vi "Get_Preset_File.vi"() -> ()   [LabVIEW 2020]
uses:
  Shared/MySQL/Preset Query Enum.ctl
panel:
  in  "Tab Control":enum32{" MAIN", "Page 2"}(tab)
  in  "Upload as Preset":bool
  in  "Preset Menu":u16(ring) items=["None", "Pulsed Alignment", "3J", "Diode", "26J", "SingleShot", "1Hz", "800 MAX ND", "Amp3-8J-CapExit", "SDI", "CapInHexPosition", "CapOutHexFiberPosition", "Full Heater, Frog Out", "Full Heater, Frog In", "MagSpecSimulateBoff", "Pulsed", "CW", "Amp2, Clunker In", "Amp3-17J", "MagSpecSimulateBon", "SMFiber-In", "SMFiber-Out", "Amp3-MegaAttenuator", "developer"]
  in  "View Preset":bool
  in  "Load ECS to Table":bool
  in  "file (use dialog)":path
  in  "Table Control":string[][](table)
  in  "Choose Values":bool
  in  "EXIT":bool
  in  "Left Join":bool
  out "PRESET FROM DB":string[][](table)
  out "ECS File":string[][](table)
  out "Coordinate Array":i32[][](array[numeric])
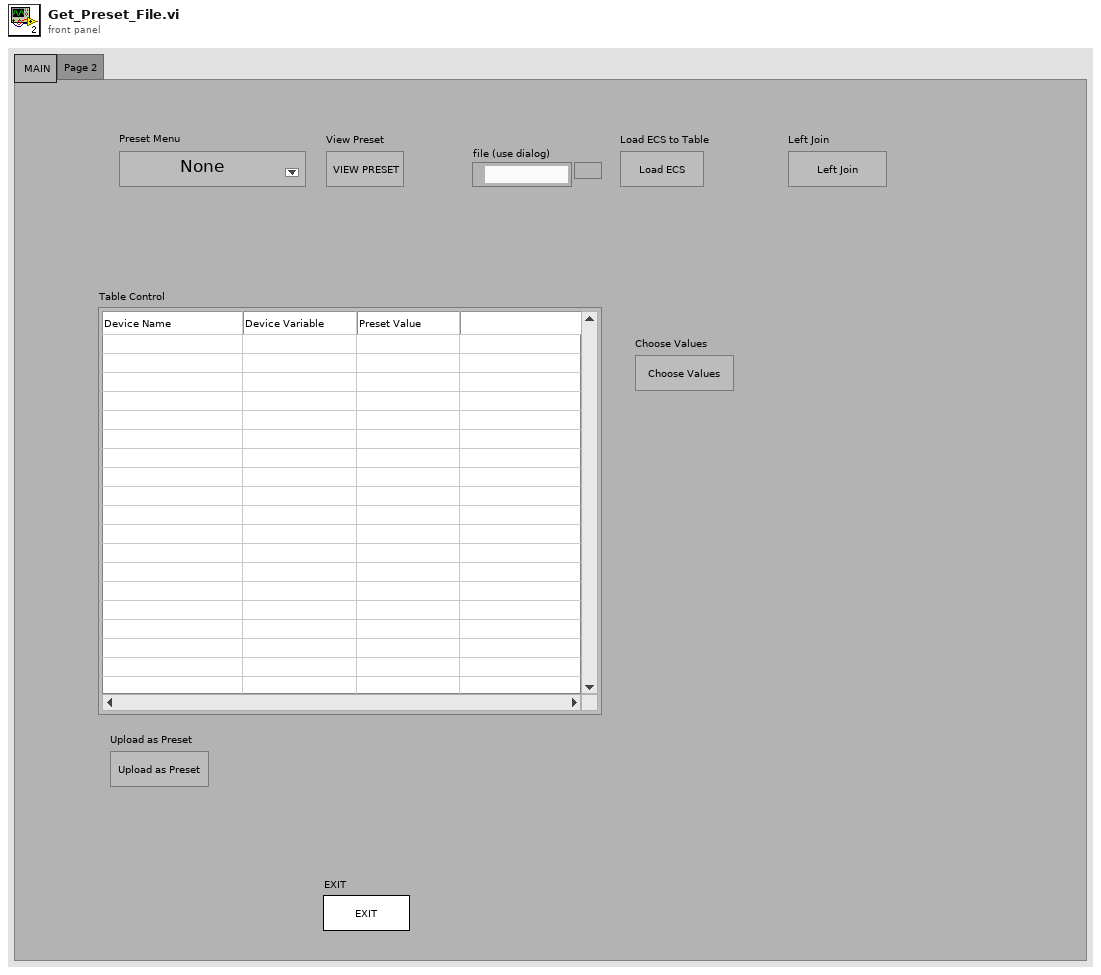
[diagram p1: front panel]
types:
  T1 = typedef "Preset Query Enum.ctl" = enum16{"Get Locations", "Get all IPs and MACs", "Get classes", "Get expt variables to set at scanstart for particular device", "Get expt devices and variables with start values", "Get expt devices and variables (with data to get)", "Get expt devices with data to get", "Get Expt devices and GUIs", "Get all devices basic properties", "Get Virtual Devices Core Info", "Get Expt names", "Get experiment basic properties", "Get experiment alarm variables", "Get MC Ports", "Get device network comm port", "Get devicetype lvclass path", "Get basic device properties", "Get Init Order", "Get all setable variables of a device", "Get device variable aliases", "Get force values of all settable variables", "Get all variables of a devicetype", "Get all variables of a device", "Get plotter details", "Get Saved Scans", "Get Scan Info", "GetGeneralGUIs", "Get expt for plotter", "Get plotter IDs from expt", "Get all devices", "Get all Virtual Devices", "Get all aliases", "Get variable and device info for Virtual Device", "GetItemLocatorIP", "Get IPs for GUIs", "Get DeviceType from Device", "GetLocalPortRange", "GetDevicePresetVariables", "Get Device Configuration", "GetAllPresetNames", "GetAllConfigurationNames", "GetPresetDeviceNames", "GetDeviceAliases", "GetDevicesOfClass"}
  T2 = enum32{"Invalid", "Standard", "Closed", "Hidden", "Minimized", "Maximized"}
  T3 = enum32{"invalid app kind", "Development System", "Run Time System", "Student Edition", "Embedded LabVIEW", "Evaluation", "Custom"}
  T4 = cluster{"Core":cluster{"Current VI Reference":refnum<vi>, "Close Panel on Exit?":bool}, "Your Boolean data":bool, "Your string data":string, "Table Control":string[][], "Column Headers[]":string[], "Temporary Preset":string[][]}
  T5 = cluster{"Current VI Reference":refnum<vi>, "Close Panel on Exit?":bool}
  T6 = enum16{"Left Button", "Center Button", "Right Button", "Window Close"}
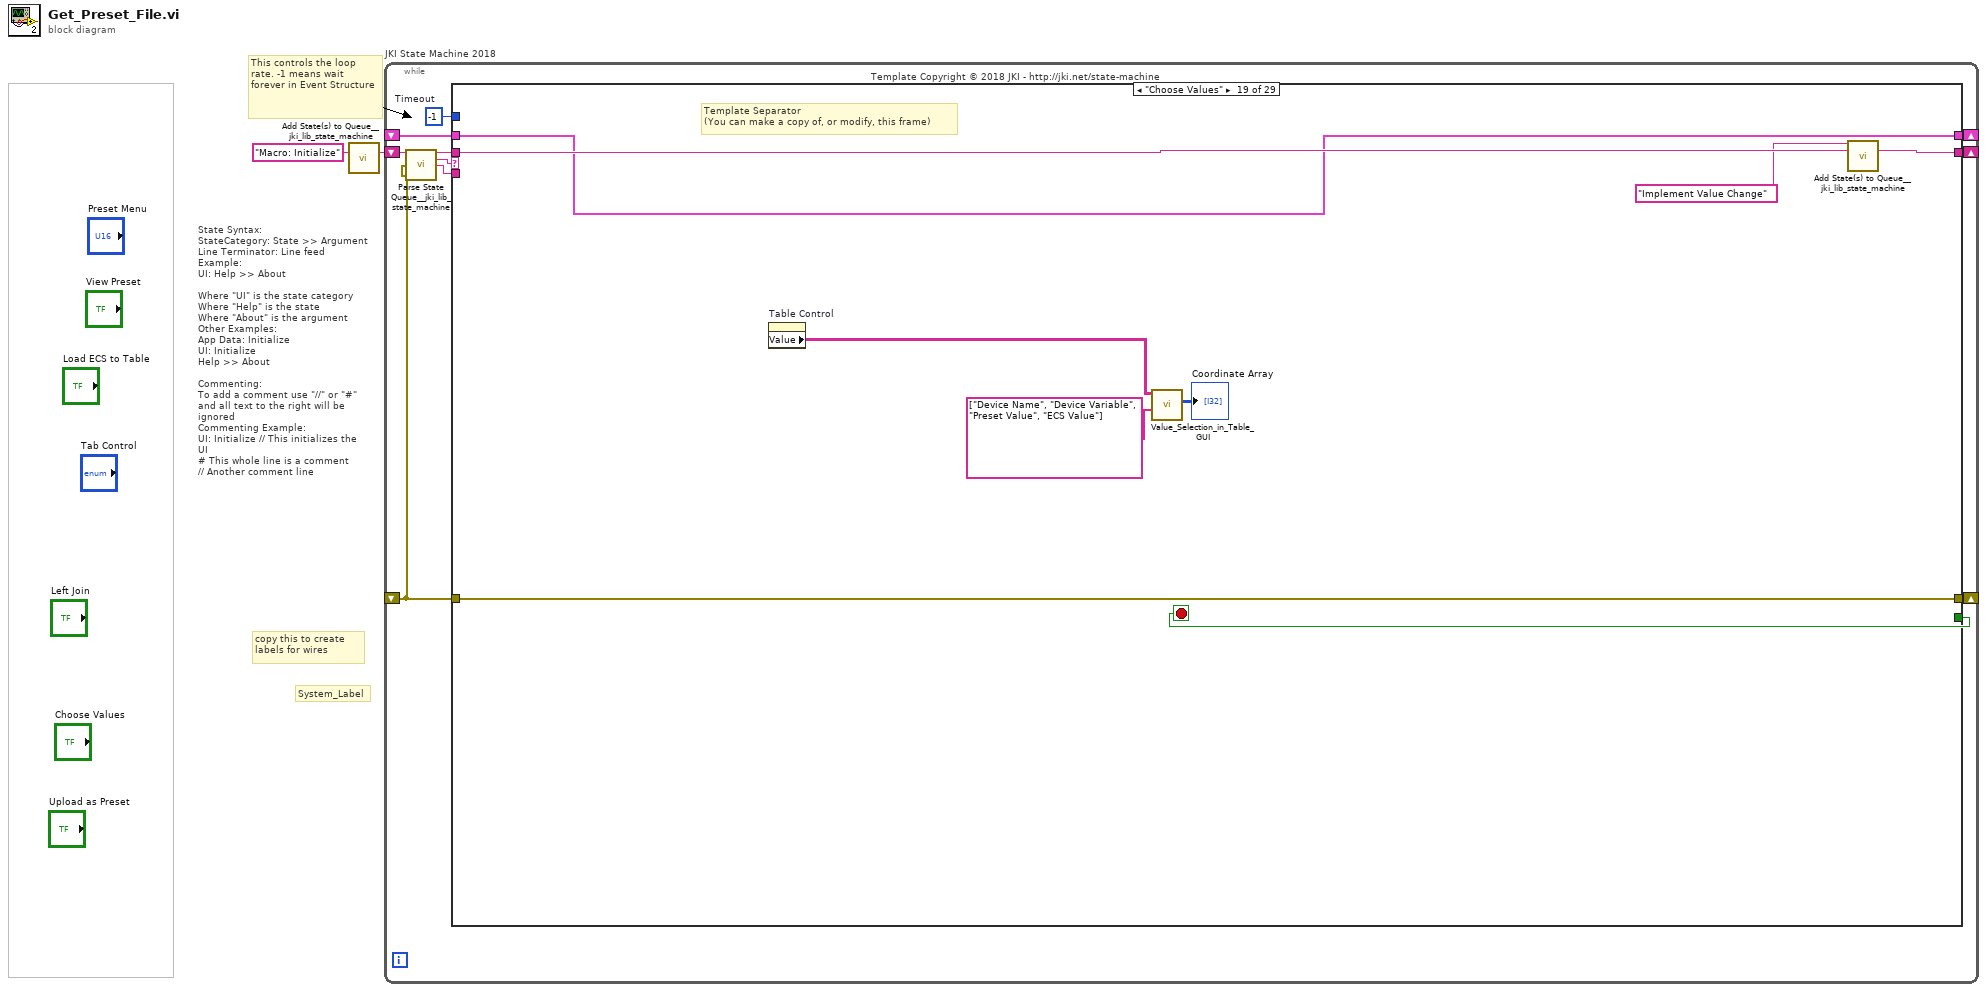
[diagram p0: block diagram]
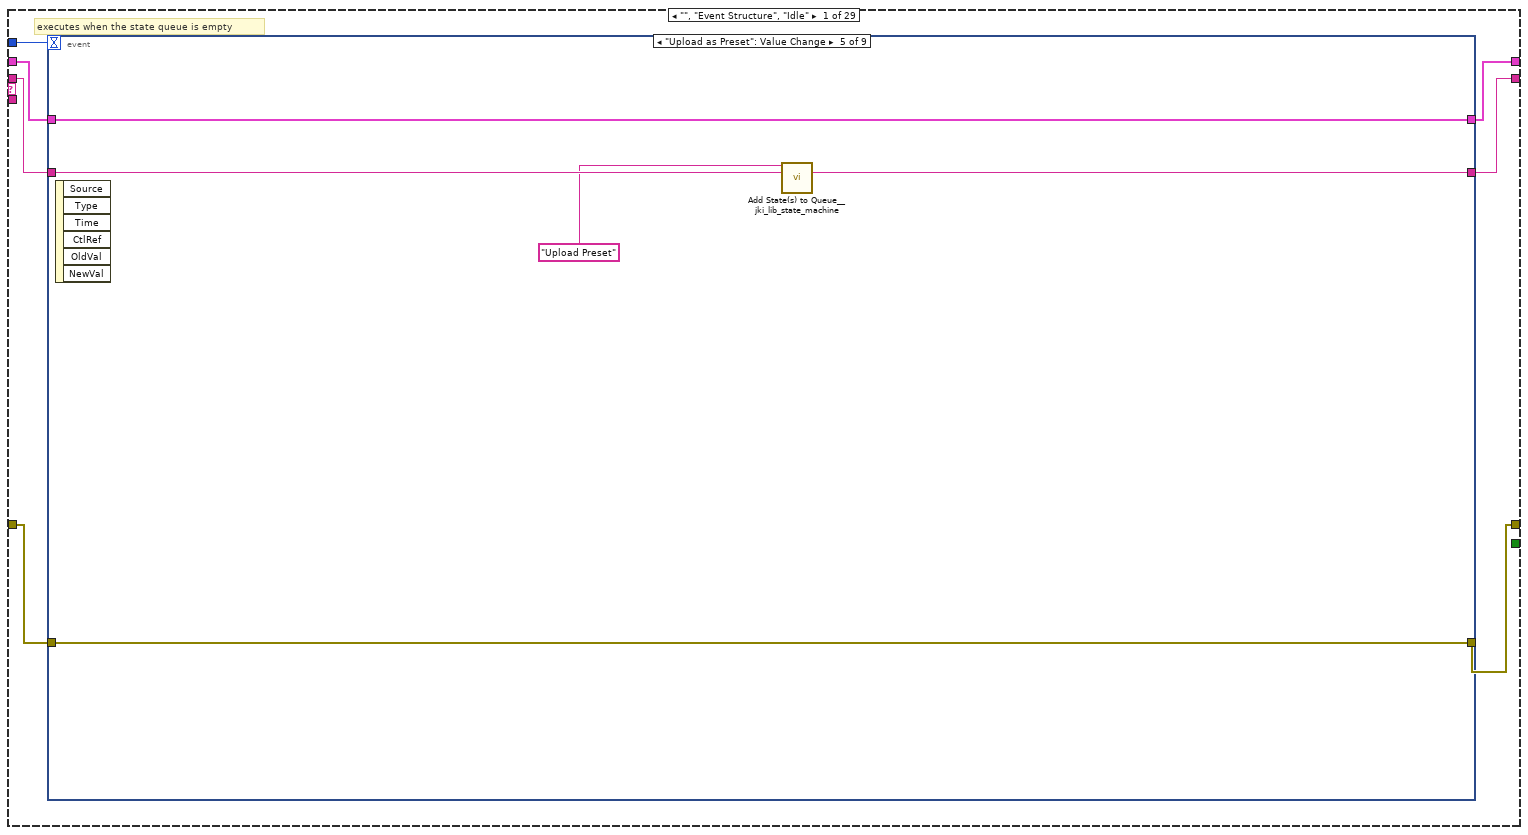
[diagram p2: hidden frame]
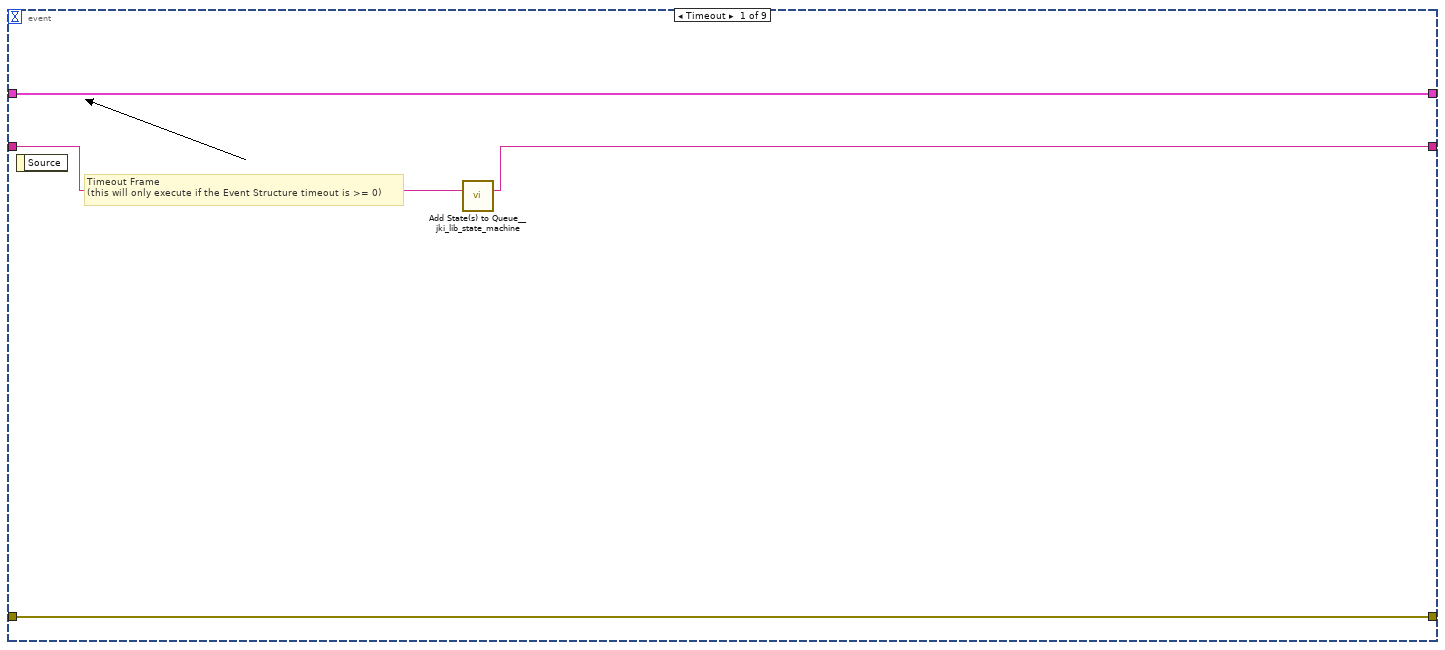
[diagram p3: hidden frame]
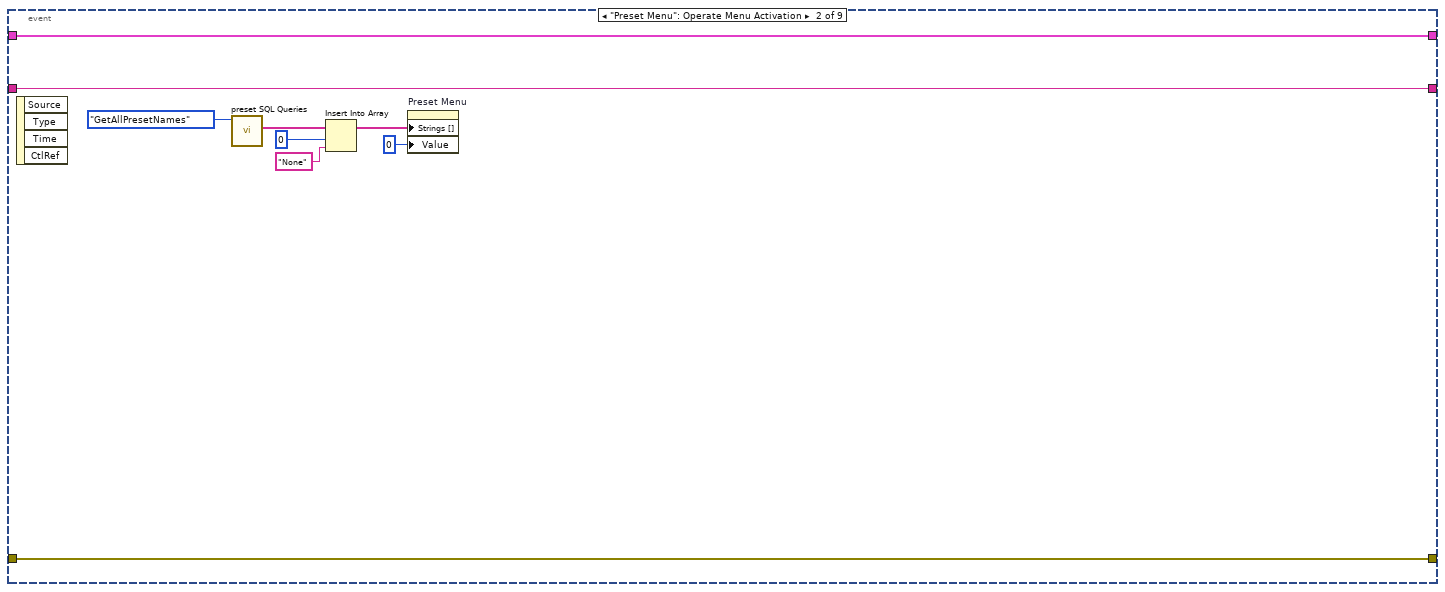
[diagram p4: hidden frame]
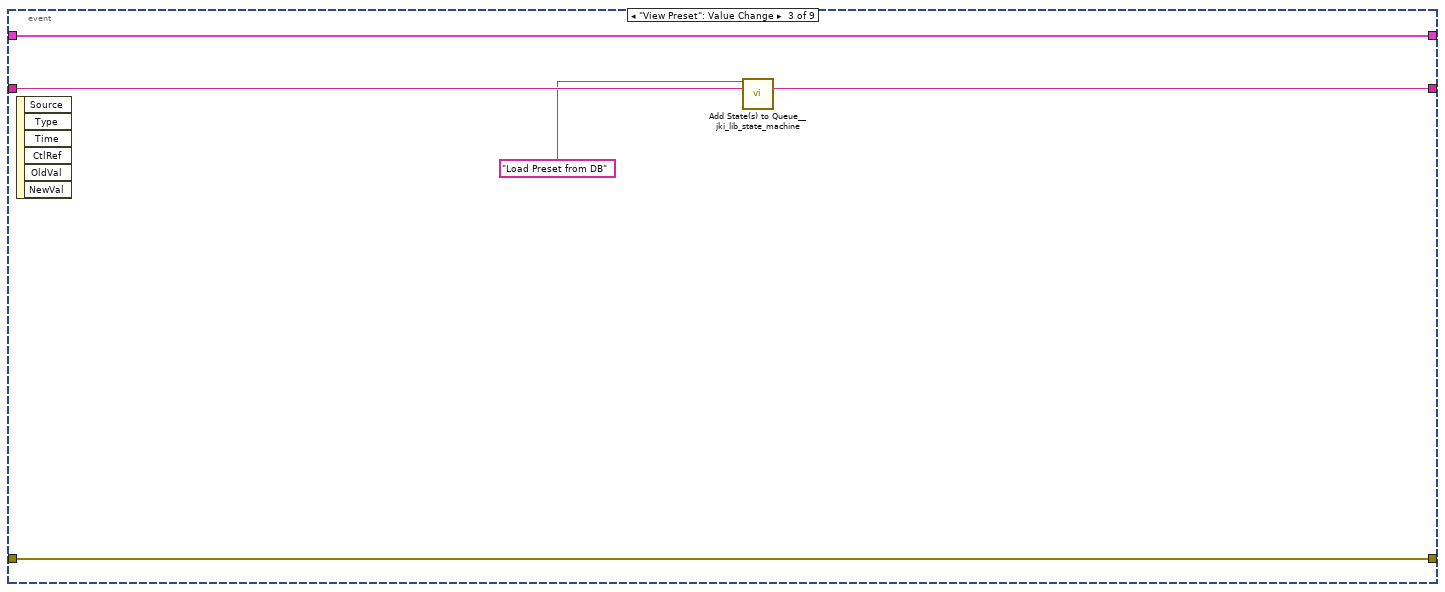
[diagram p5: hidden frame]
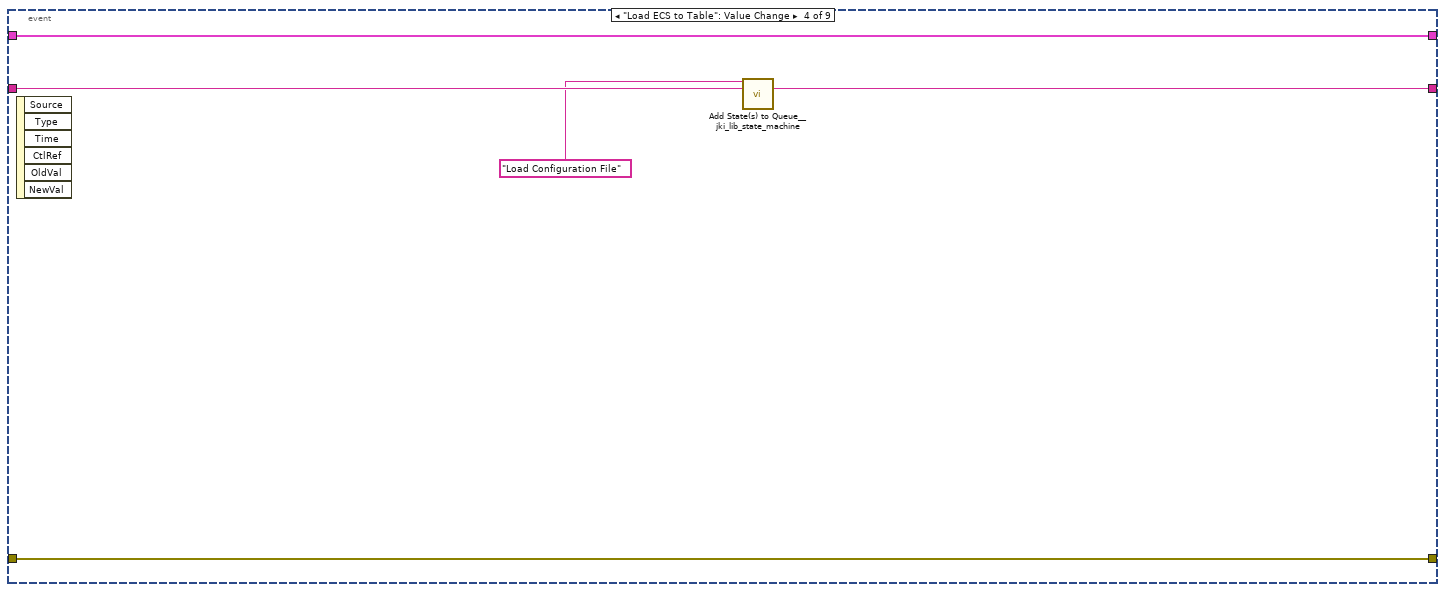
[diagram p6: hidden frame]
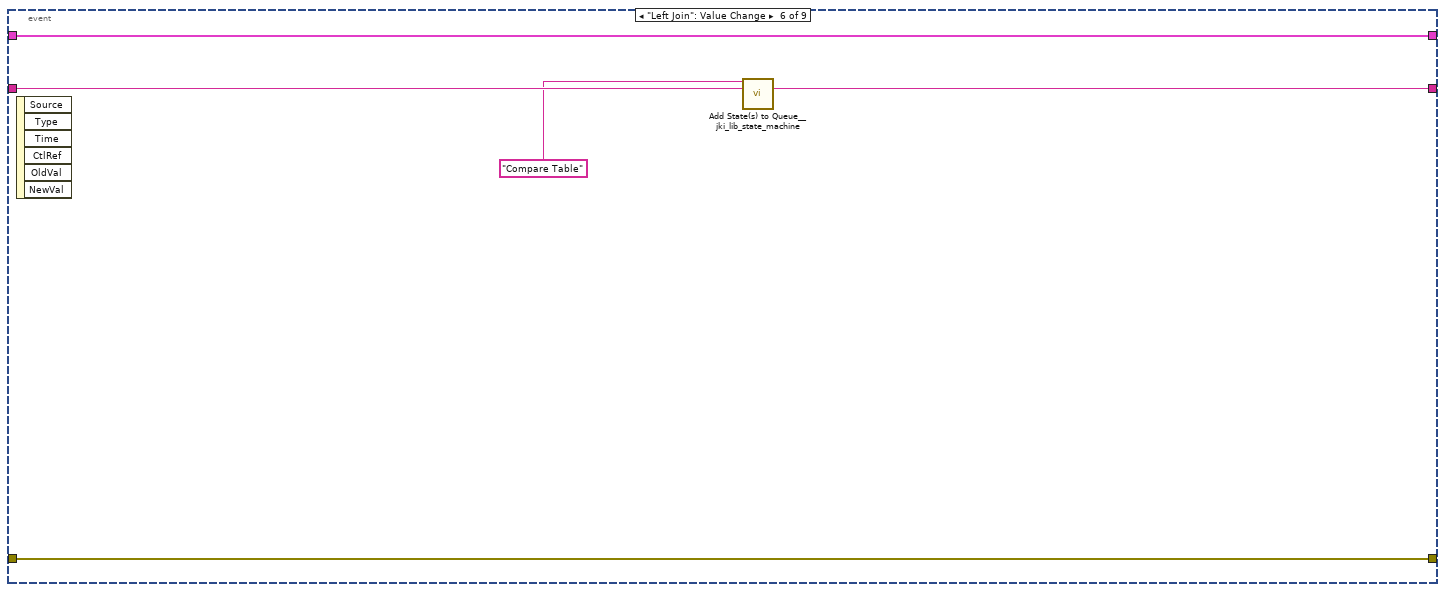
[diagram p7: hidden frame]
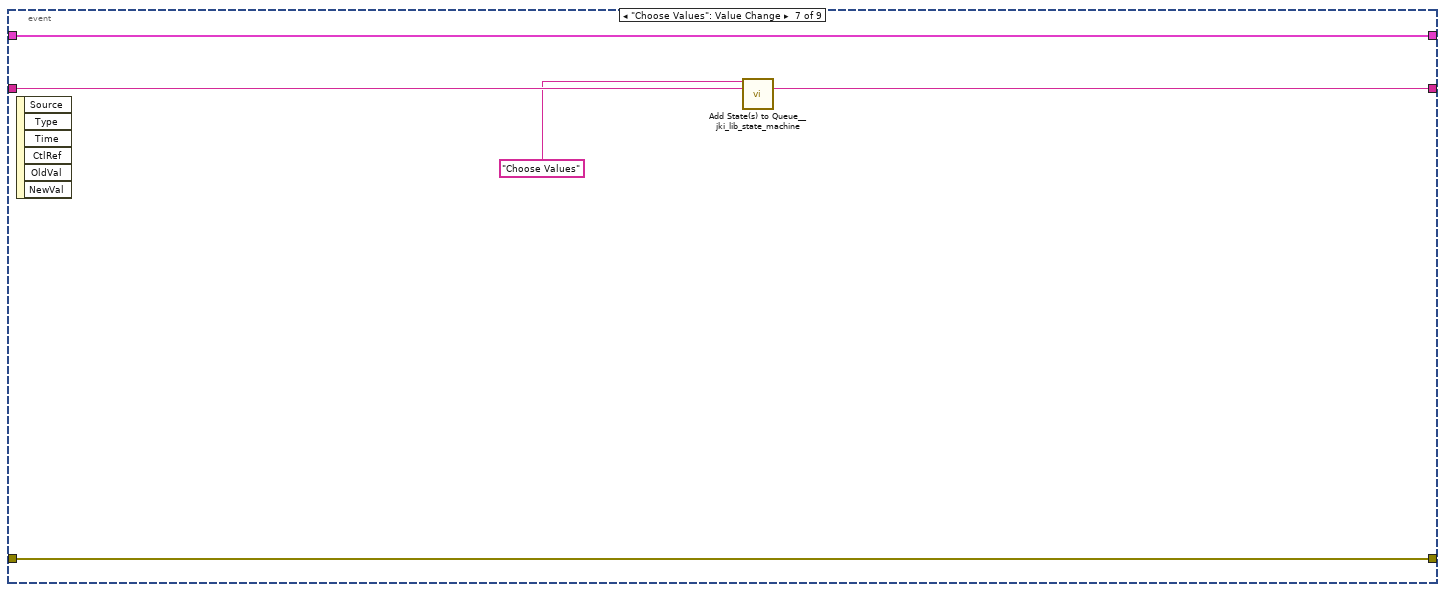
[diagram p8: hidden frame]
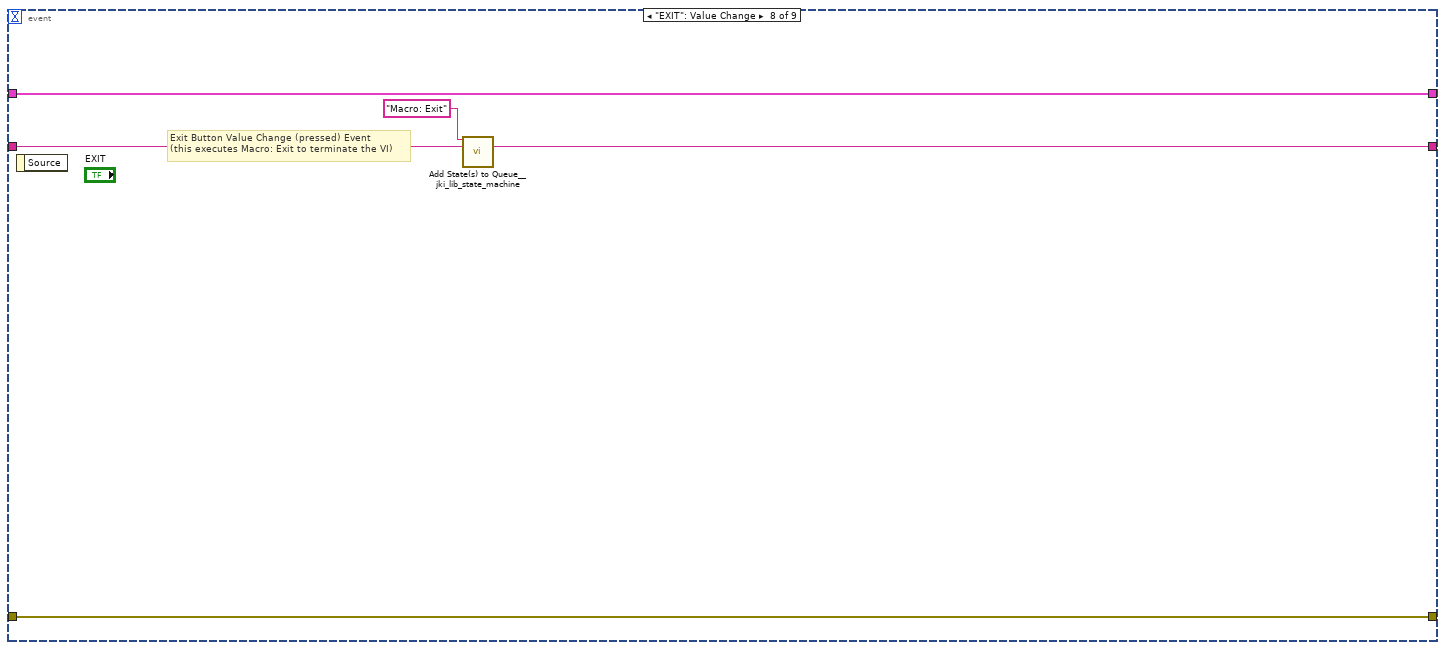
[diagram p9: hidden frame]
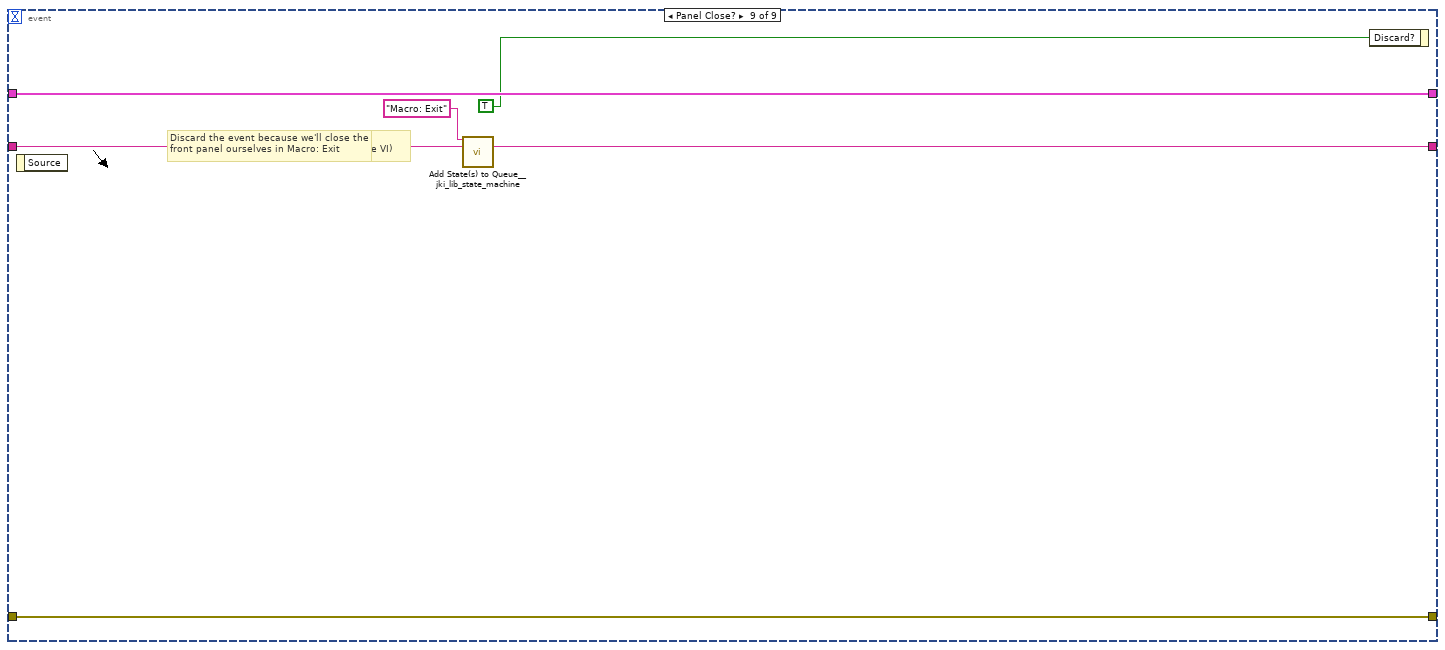
[diagram p10: hidden frame]
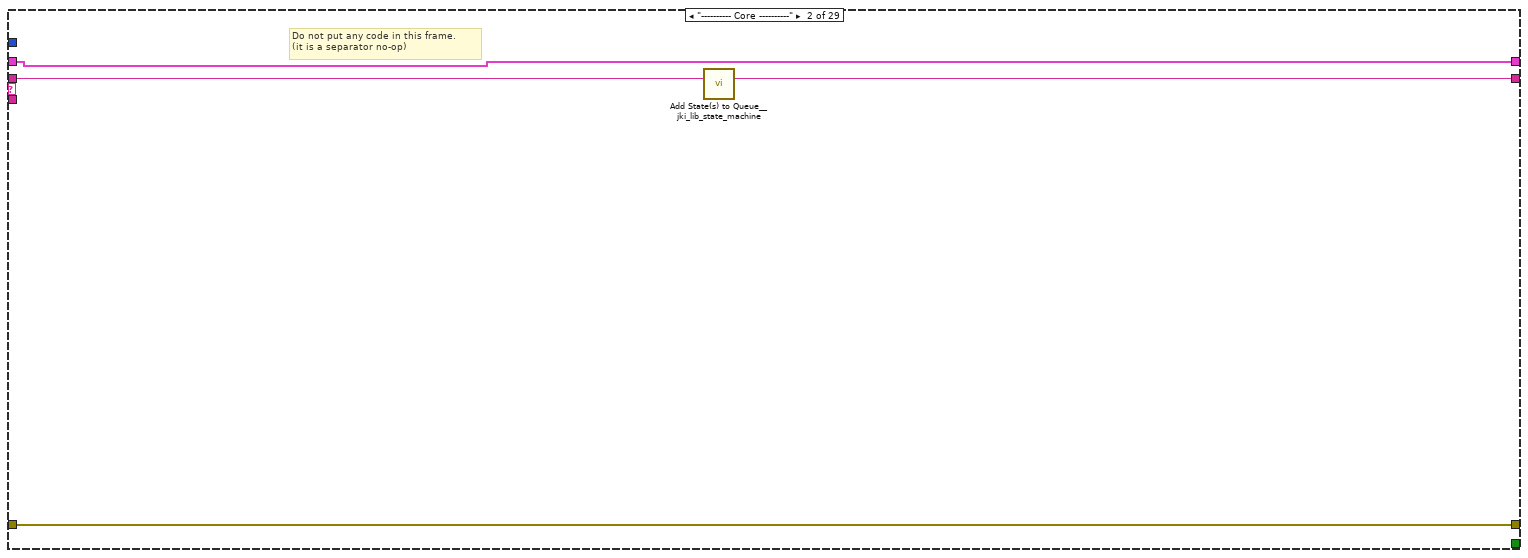
[diagram p11: hidden frame]
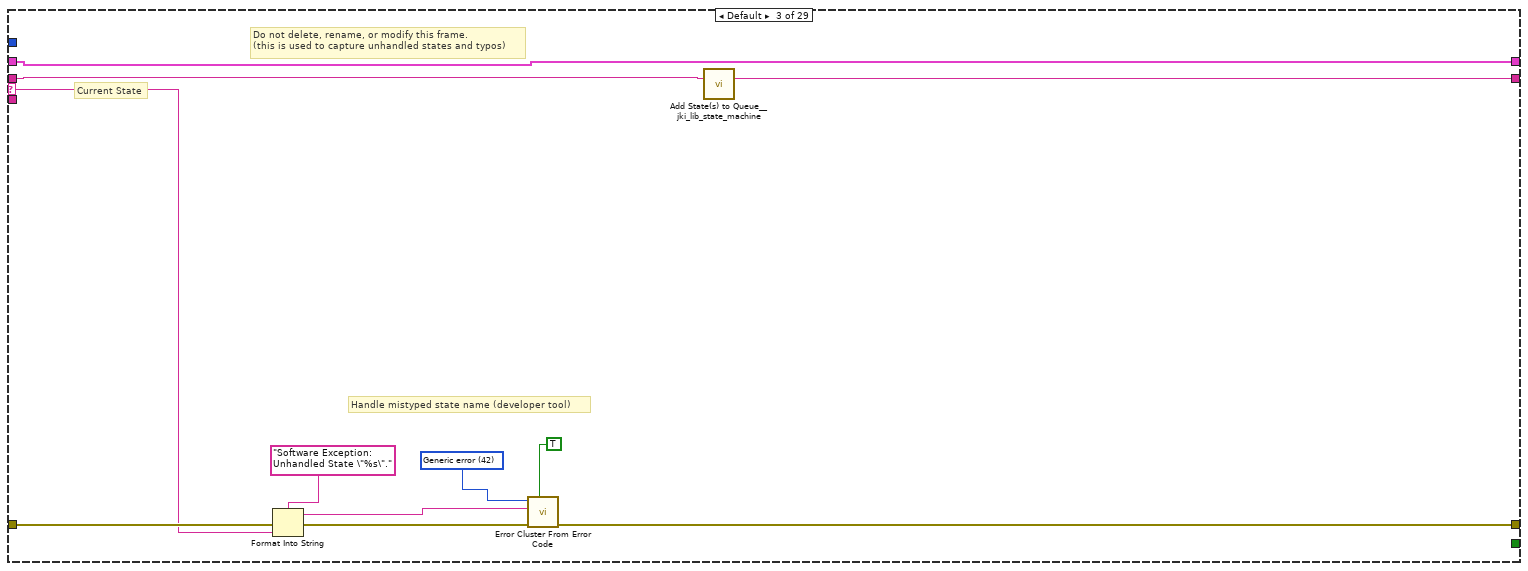
[diagram p12: hidden frame]
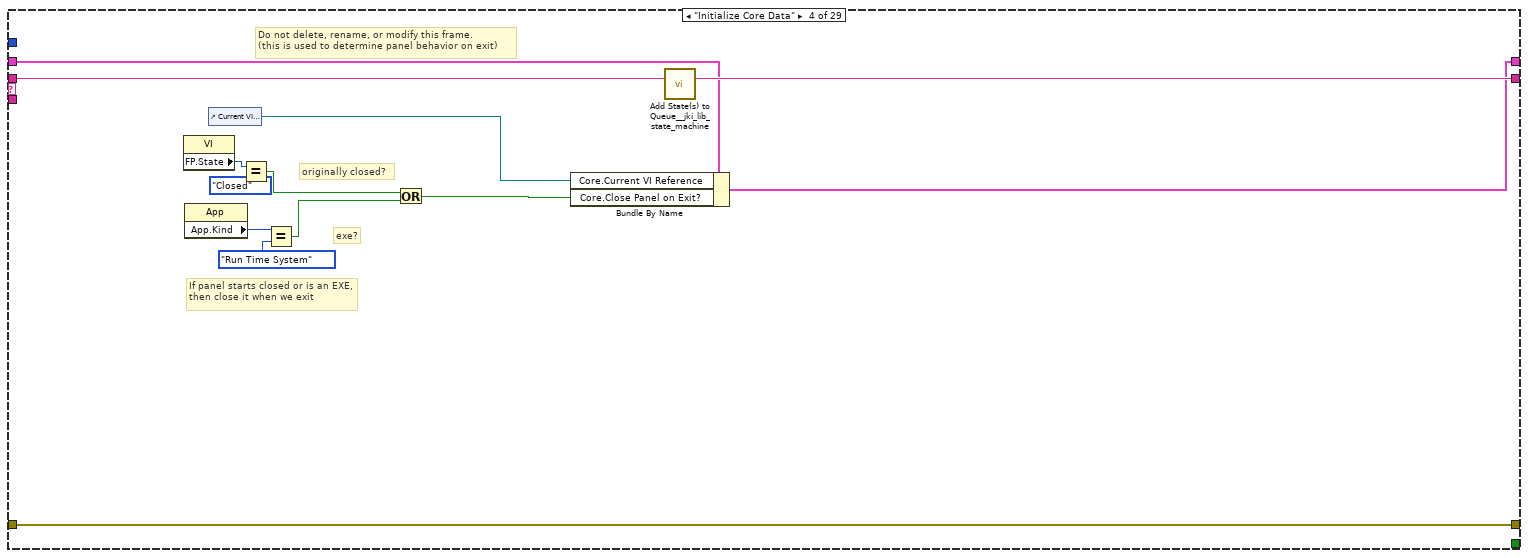
[diagram p13: hidden frame]
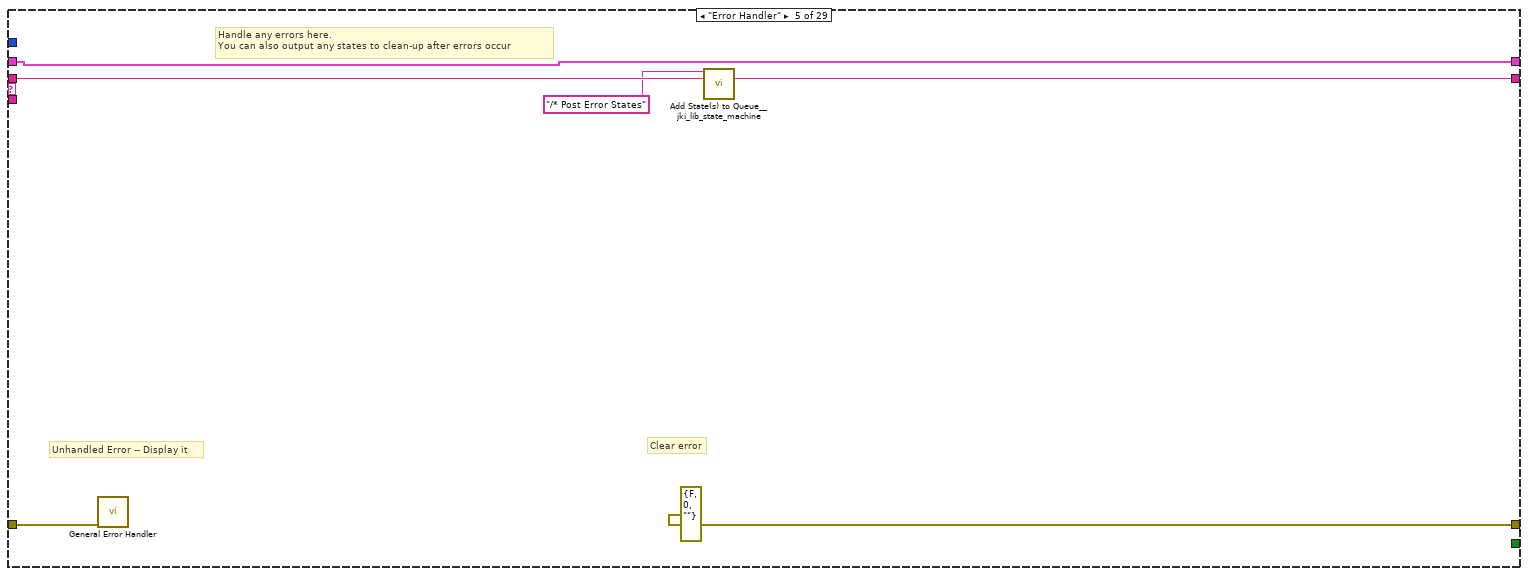
[diagram p14: hidden frame]
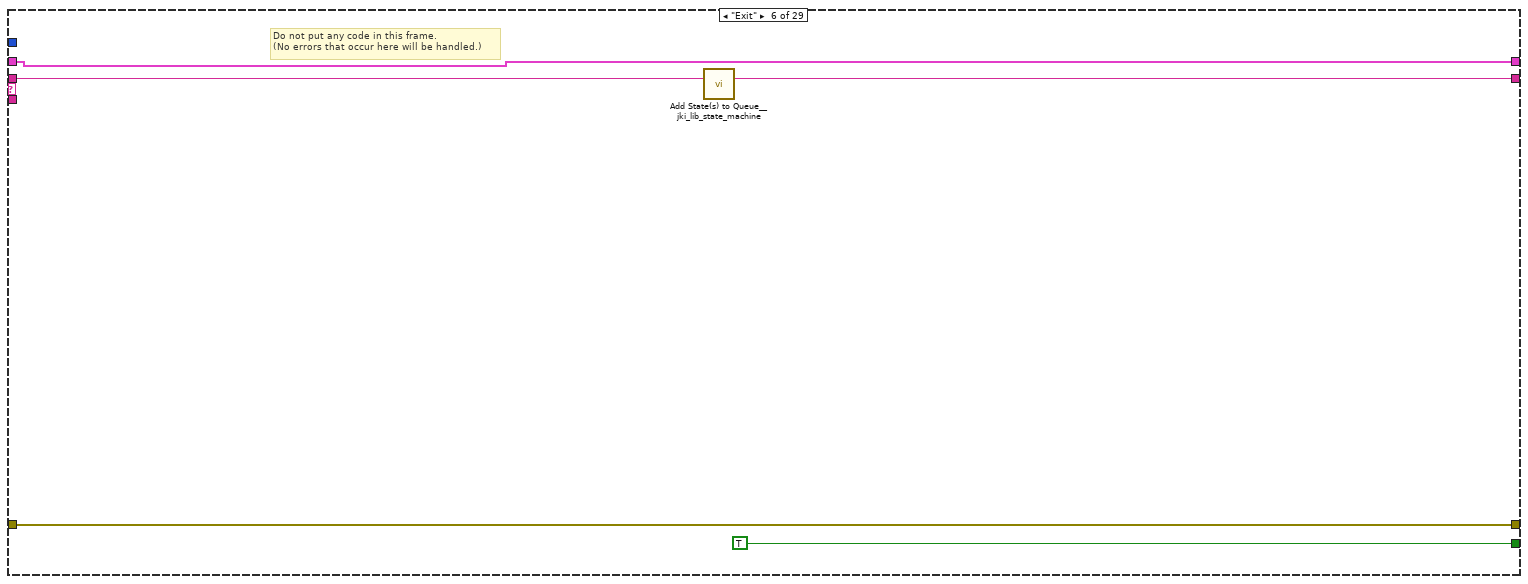
[diagram p15: hidden frame]
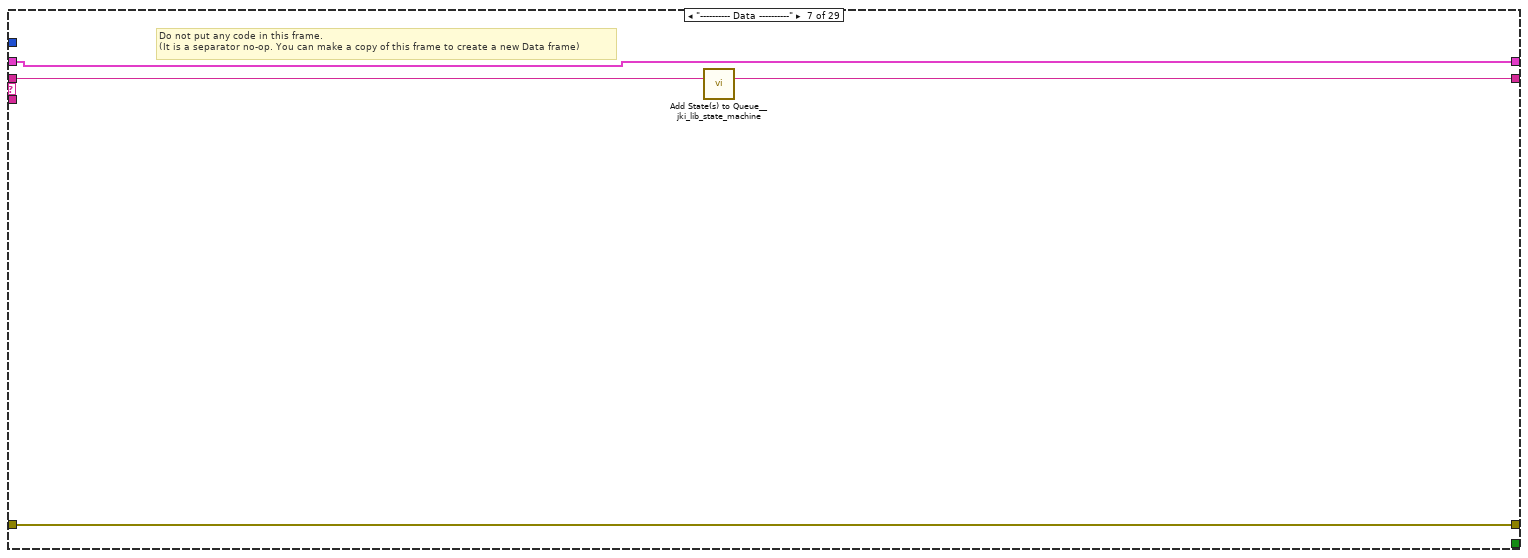
[diagram p16: hidden frame]
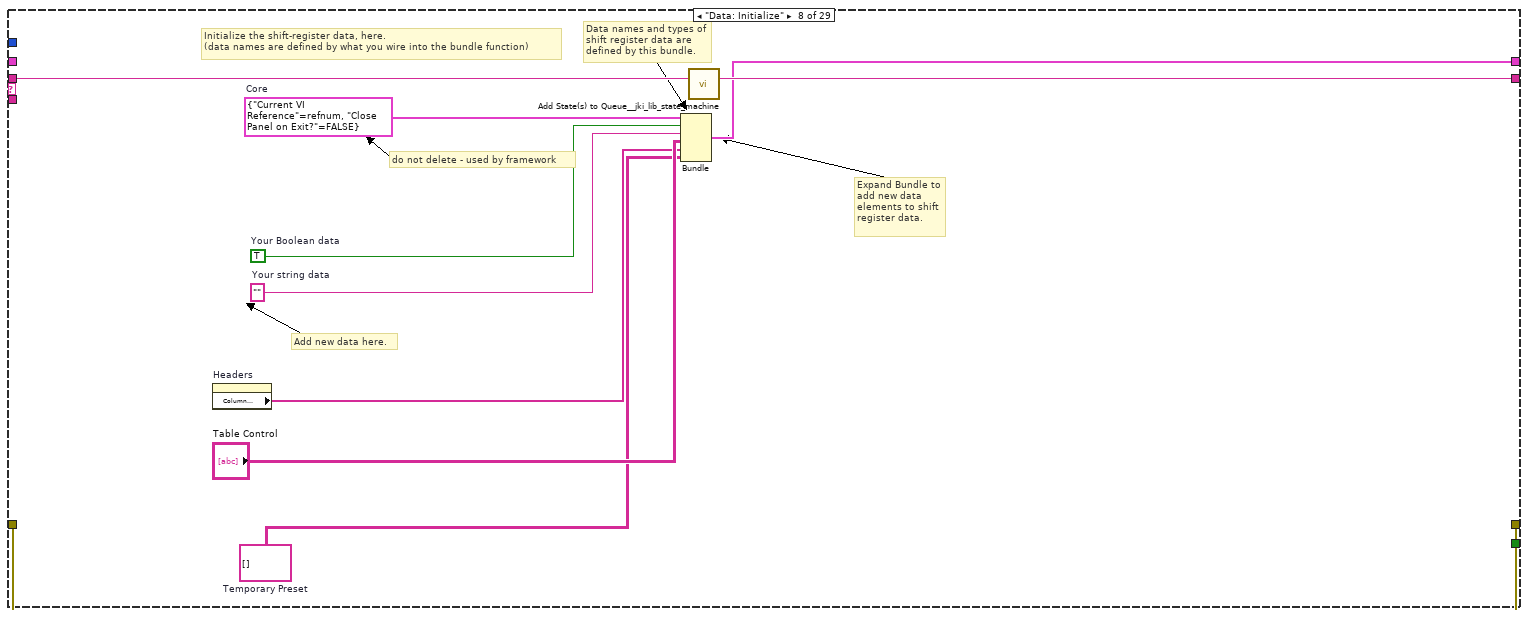
[diagram p17: hidden frame]
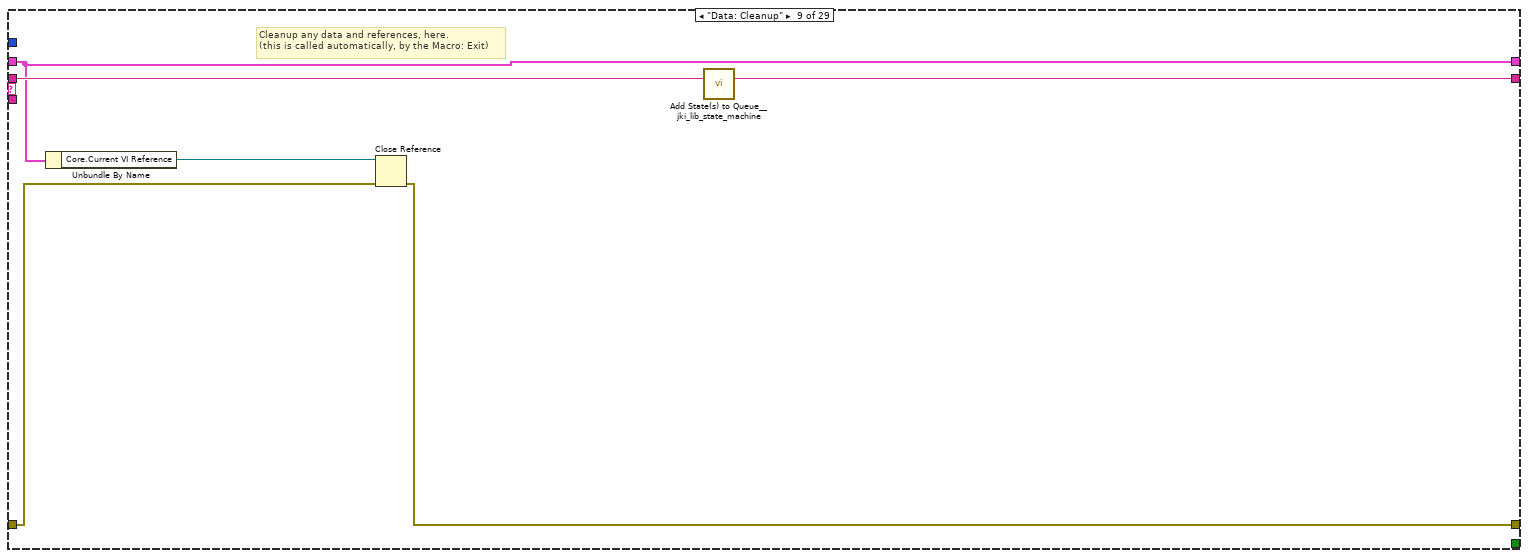
[diagram p18: hidden frame]
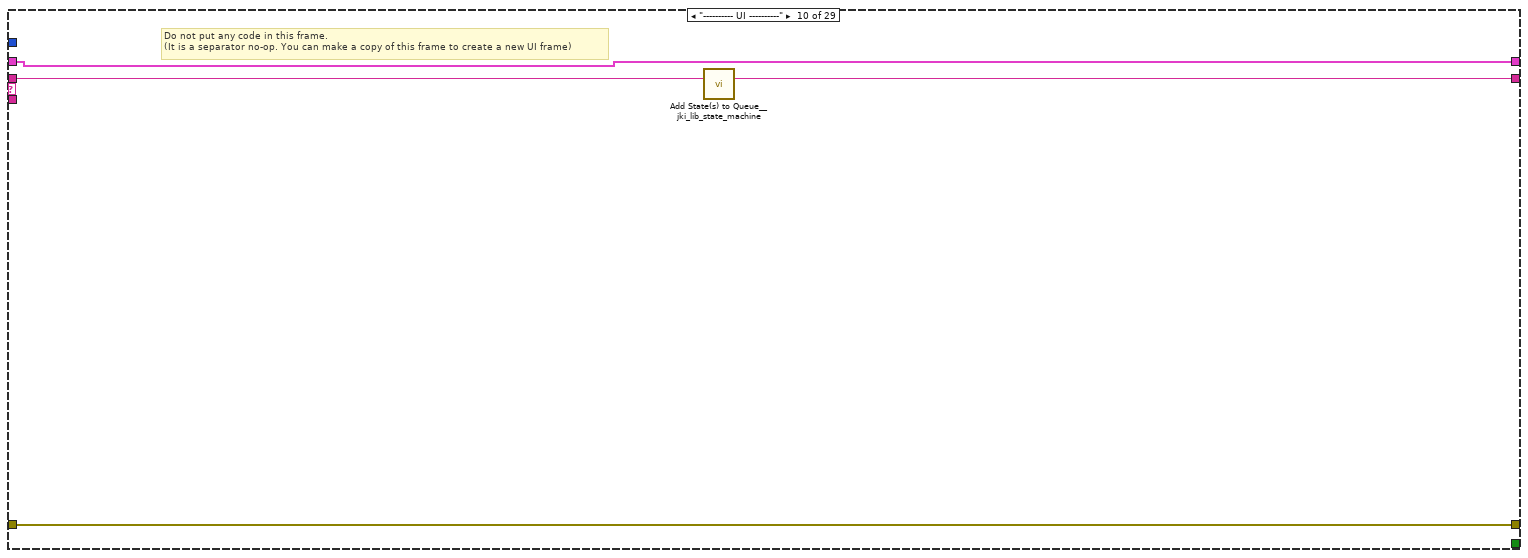
[diagram p19: hidden frame]
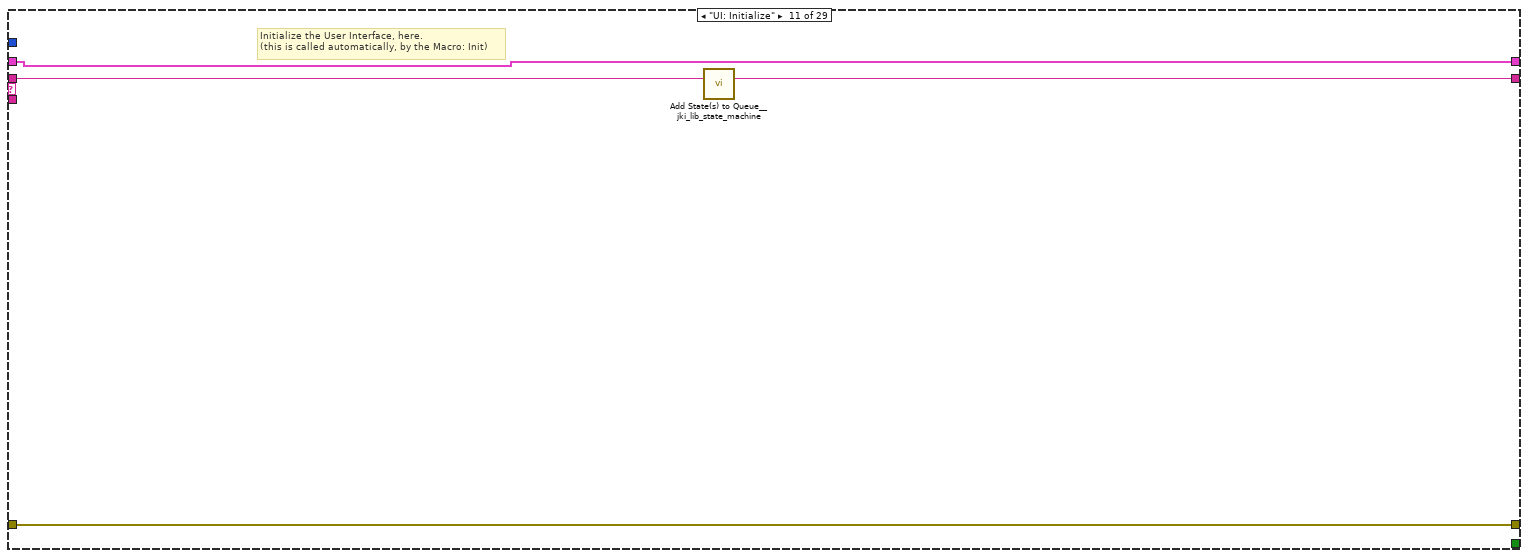
[diagram p20: hidden frame]
diagram:
  # "State Syntax:\nStateCategory: State >> Argument\nLine Terminator: Line feed\nExample:\nUI: Help >> About\n\nWhere \"UI\" is the state category\nWhere \"Help\" is the state\nWhere \"About\" is the argument\nOther Examples:\nApp Data: Initialize\nUI: Initialize\nHelp >> About\n\nCommenting:\nTo add a comment use \"//\" or \"#\" and all text to the right will be ignored\nCommenting Example:\nUI: Initialize // This initializes the UI\n# This whole line is a comment\n// Another comment line"
  # "copy this to create labels for wires"
  # "This controls the loop rate. -1 means wait forever in Event Structure"
  # "System_Label"
  n1 = call <vilib>:"Add State(s) to Queue__jki_lib_state_machine.vi"("State(s) in (\"\")"="Macro: Initialize") -> ("States Out"=w2:string)  [unwired: 14 in]
  n2 = while "JKI State Machine 2018" {
    shift-right: [w6] -> _
    shift-left: _ -> [w5]
    shift-right: [w9] -> _
    shift-left: _ -> [w3]
    shift-right: [w8] -> _
    shift-left: w2 -> [w10]
    stop <- w7 stop-if-true
    w4 = -1  # Timeout
    # "Template Copyright © 2018 JKI - http://jki.net/state-machine"
    n3 = call <vilib>:"Parse State Queue__jki_lib_state_machine.vi"("State Queue"=w10, "Error In (no error)"=w3) -> ("Remaining States"=w12:string, "Current State"=w13:string, "Arguments"=w11:string)  [unwired: 11 in]
    n4 = case shown="\"Choose Values\"" w13 {
      selector: w13 -> [_ _ w74 _ _ _ _ _ _ _ _ _ _ _ _ _ _ _ _ _ _ _ _ _ _ _ _ _ _]
      tunnel: w12 -> [w20 w73 w78 w97 w103 w108 w112 w122 w128 w132 w136 w142 w153 w222 w227 w237 w241 w251 w259 w269 w282 w307 w317 w334 w347 w351 w355 w359 w365]
      tunnel: w11 -> [_ _ _ _ _ _ _ _ _ _ _ w137 w147 _ _ _ _ _ _ _ _ _ _ _ _ _ _ _ _]
      tunnel: w5 -> [w18 w70 w76 w90 w100 w106 w109 _ w123 w129 w134 w140 w149 w219 w224 w234 w238 w246 w252 w265 w274 w303 w314 w330 w343 w348 w352 w356 w362]
      tunnel: [w17 w71 w80 w94 errorcluster {"status"=FALSE, "code"=0, "source"=""} ("error out") w105 w110 w120 w124 w130 w133 w138 w150 w220 w225 w235 w239 w249 w257 w267 w280 w305 w315 w332 w345 w349 w353 w357 w363] -> w9
      tunnel: w3 -> [w16 w71 w79 w94 w99 w105 w110 w120 w125 w130 w133 w139 w151 w220 w225 w235 w239 w249 w257 w267 w280 w305 w315 w332 w345 w349 w353 w357 w363]
      tunnel: [w19 w72 w77 w96 w102 w107 w111 w121 w127 w131 w135 w141 w152 w221 w226 w236 w240 w250 w258 w268 w281 w306 w316 w333 w346 w350 w354 w358 w364] -> w8
      tunnel: [_ _ _ _ _ TRUE _ _ _ _ _ _ _ _ _ _ _ _ _ _ _ _ _ _ _ _ _ _ _] -> w7
      tunnel: [w15 w70 w76 w95 w100 w106 w109 w116 w123 w129 w134 w140 w149 w219 w224 w234 w238 w244 w252 w264 w273 w302 w314 w330 w343 w348 w352 w356 w362] -> w6
      tunnel: w4 -> [w14 _ _ _ _ _ _ _ _ _ _ _ _ _ _ _ _ _ _ _ _ _ _ _ _ _ _ _ _]
      frame "", "Event Structure", "Idle" {
        # "executes when the state queue is empty"
        n5 = event shown="[4] \"Upload as Preset\": Value Change" {
          selector: _ -> [_ _ _ _ _ _ _ _ _]
          dyn-events: _ -> [_ _ _ _ _ _ _ _ _]
          timeout: w14 -> [_ _ _ _ _ _ _ _ _]
          tunnel: w20 -> [w24 w32 w36 w41 w46 w51 w56 w63 w69]
          tunnel: [w23 w32 w35 w40 w45 w50 w55 w62 w68] -> w19
          tunnel: w18 -> [w21 w33 w38 w43 w48 w53 w58 w60 w66]
          tunnel: [w22 w31 w37 w42 w47 w52 w57 w61 w67] -> w17
          tunnel: w16 -> [w22 w31 w37 w42 w47 w52 w57 w61 w67]
          tunnel: [w21 w33 w38 w43 w48 w53 w58 w60 w66] -> w15
          event Timeout {
            # "Timeout Frame\n(this will only execute if the Event Structure timeout is >= 0)"
            n6 = event-data() -> ()  [unwired: 1 in, 1 out]
            n7 = call <vilib>:"Add State(s) to Queue__jki_lib_state_machine.vi"("State(s) in (\"\")"=w24) -> ("States Out"=w23:string)  [unwired: 14 in]
          }
          event "Preset Menu": Operate Menu Activation {
            n8 = event-data() -> ()  [unwired: 1 in, 4 out]
            n9 = call "preset SQL Queries.vi"("Preset Query"=Preset_Query_Enum."GetAllPresetNames") -> ("1st column 1st data"=w29:string[])  [unwired: 8 in, 2 out]
            n10 = Insert Into Array(array=w29, index=0, new element="None" ("new element/subarray")) -> (w26:string[])
            n11 = property on="Preset Menu" class="Ring (strict)"("Strings []"=w26, "Value"=0 ("index")) -> ()  [unwired: 2 in, 2 out]
          }
          event "View Preset": Value Change {
            n12 = event-data() -> ()  [unwired: 1 in, 6 out]
            n13 = call <vilib>:"Add State(s) to Queue__jki_lib_state_machine.vi"("State(s) in Front (\"\")"="Load Preset from DB", "State(s) in (\"\")"=w36) -> ("States Out"=w35:string)  [unwired: 13 in]
          }
          event "Load ECS to Table": Value Change {
            n14 = event-data() -> ()  [unwired: 1 in, 6 out]
            n15 = call <vilib>:"Add State(s) to Queue__jki_lib_state_machine.vi"("State(s) in Front (\"\")"="Load Configuration File", "State(s) in (\"\")"=w41) -> ("States Out"=w40:string)  [unwired: 13 in]
          }
          event "Upload as Preset": Value Change {
            n16 = event-data() -> ()  [unwired: 1 in, 6 out]
            n17 = call <vilib>:"Add State(s) to Queue__jki_lib_state_machine.vi"("State(s) in Front (\"\")"="Upload Preset", "State(s) in (\"\")"=w46) -> ("States Out"=w45:string)  [unwired: 13 in]
          }
          event "Left Join": Value Change {
            n18 = event-data() -> ()  [unwired: 1 in, 6 out]
            n19 = call <vilib>:"Add State(s) to Queue__jki_lib_state_machine.vi"("State(s) in Front (\"\")"="Compare Table", "State(s) in (\"\")"=w51) -> ("States Out"=w50:string)  [unwired: 13 in]
          }
          event "Choose Values": Value Change {
            n20 = event-data() -> ()  [unwired: 1 in, 6 out]
            n21 = call <vilib>:"Add State(s) to Queue__jki_lib_state_machine.vi"("State(s) in Front (\"\")"="Choose Values", "State(s) in (\"\")"=w56) -> ("States Out"=w55:string)  [unwired: 13 in]
          }
          event "EXIT": Value Change {
            # "Exit Button Value Change (pressed) Event\n(this executes Macro: Exit to terminate the VI)"
            n22 = event-data() -> ()  [unwired: 1 in, 1 out]
            n23 = call <vilib>:"Add State(s) to Queue__jki_lib_state_machine.vi"("State(s) in Front (\"\")"="Macro: Exit", "State(s) in (\"\")"=w63) -> ("States Out"=w62:string)  [unwired: 13 in]
          }
          event Panel Close? {
            # "Discard the event because we'll close the front panel ourselves in Macro: Exit"
            # "Close Panel button (pressed) Event\n(this executes Macro: Exit to terminate the VI)"
            n24 = event-data() -> ()  [unwired: 1 in, 1 out]
            n25 = call <vilib>:"Add State(s) to Queue__jki_lib_state_machine.vi"("State(s) in Front (\"\")"="Macro: Exit", "State(s) in (\"\")"=w69) -> ("States Out"=w68:string)  [unwired: 13 in]
            n26 = event-data("Discard?"=TRUE) -> ()  [unwired: 1 in, 1 out]
          }
        }
      }
      frame "---------- Core ----------" {
        # "Do not put any code in this frame.\n(it is a separator no-op)"
        n27 = call <vilib>:"Add State(s) to Queue__jki_lib_state_machine.vi"("State(s) in (\"\")"=w73) -> ("States Out"=w72:string)  [unwired: 14 in]
      }
      frame Default {
        w83 = 42 items=["No error", "Argument error", "Memory is full", "Out of zone", "End of file", "File already open", "Generic file I/O error", "File not found", "File permission error", "Disk is full", "Duplicate path", "Too many files open", "System feature not enabled", "Resource file not found", "Cannot add resource", "Resource not found", "Image not found", "Image memory error", "Pen does not exist", "Config type invalid", "Config token not found", "Config parse error", "Config memory error", "Bad external code format", "Bad external code offset", "External code not present", "Null window", "Destroy window error", "Null menu", "Print aborted", "Bad print record", "Print driver error", "Windows error during printing", "Memory error during printing", "Print dialog error", "Generic print error", "Invalid device refnum", "Device not found", "Device parameter error", "Device unit error", "Cannot open device", "Device call aborted", "Generic error", "Cancelled by user", "Object ID too low", "Object ID too high", "Object not in heap", "Unknown heap", "Unknown object (invalid DefProc)", "Unknown object (DefProc not in table)", "Message out of range", "Invalid (null) method", "Unknown message", "Manager call not supported", "Bad address", "Network operation in progress", "Network operation timed out", "Connection is busy", "Network attribute not supported", "Network error", "Address in use", "System out of memory", "Connection aborted", "Connection refused", "Not connected", "Already connected", "Connection closed", "Initialization error (interapplication manager)", "Bad occurrence", "Wait on unbound occurrence handler", "Occurrence queue overflow", "Datalog type conflict", "Unused", "Unrecognized type (interapplication manager)", "Memory corrupt", "Failed to make temporary DLL", "Old CIN version", "Drag socket not found", "Failed to load drop-object", "Failed to register OLE object", "Failed to release OLE object", "Format specifier type mismatch", "Unknown format specifier", "Too few format specifiers", "Too many format specifiers", "Scan failed", "Newer CIN version", "Error converting to variant", "Runtime menu error", "Password tampered", "Variant attribute not found", "Incompatible variant data type", "Event data is not available", "Event Store is not present", "Occurrence is not found", "Event Queue is not created", "Event info is not available", "Refnum passed is NULL", "Error retrieving Class GUID", "Error retrieving CoClass GUID", "Error retrieving TypeLib GUID.", "Bad built application magic bytes.", "Specific driver is different from the specific driver associated with the Logical Name.", "There is no session opened to the class driver.", "Max Error", "MAX - Error with config objects", "MAX - Error loading configuration", "MAX - Group not supported"]
        # "Current State"
        # "Do not delete, rename, or modify this frame.\n(this is used to capture unhandled states and typos)"
        # "Handle mistyped state name (developer tool)"
        n28 = Format Into String(format string="Software Exception: Unhandled State \"%s\"." ("message"), error in=w79, w74) -> (resulting string=w82:string, error out=w81:errorcluster)  [unwired: 1 in]
        n29 = call <vilib>:"Error Cluster From Error Code.vi"("show call chain? (False)"=TRUE, "error in (no error)"=w81, "error message (\"\")"=w82, "error code (0)"=w83) -> ("error out"=w80:errorcluster)  [unwired: 5 in]
        n30 = call <vilib>:"Add State(s) to Queue__jki_lib_state_machine.vi"("State(s) in (\"\")"=w78) -> ("States Out"=w77:string)  [unwired: 14 in]
      }
      frame "Initialize Core Data" {
        # "Do not delete, rename, or modify this frame.\n(this is used to determine panel behavior on exit)"
        # "originally closed?"
        # "exe?"
        # "If panel starts closed or is an EXE, then close it when we exit"
        n31 = property class="VI"() -> ("FP.State"=w87:T2)  [unwired: 2 in, 2 out]
        n32 = property class="App"() -> ("App.Kind"=w93:T3)  [unwired: 2 in, 2 out]
        n33 = control-ref of="Current VI Reference"() -> (w88:refnum<vi>)
        n34 = Equal?(x=w87, y=T2."Closed" ("Front Panel Window:State")) -> (x = y?=w85:bool)
        n35 = Equal?(x=w93, y=T3."Run Time System" ("Application:Kind")) -> (x = y?=w91:bool)
        n36 = Or(x=w85, y=w91) -> (x .or. y?=w89:bool)
        n37 = Bundle By Name(cluster=w90, "Core.Current VI Reference"=w88, "Core.Close Panel on Exit?"=w89) -> (w95:T4)
        n38 = call <vilib>:"Add State(s) to Queue__jki_lib_state_machine.vi"("State(s) in (\"\")"=w97) -> ("States Out"=w96:string)  [unwired: 14 in]
      }
      frame "Error Handler" {
        # "Unhandled Error -- Display it"
        # "Handle any errors here.\nYou can also output any states to clean-up after errors occur"
        # "Clear error"
        n39 = call <vilib>:"General Error Handler.vi"("error in (no error)"=w99) -> ()  [unwired: 10 in, 5 out]
        n40 = call <vilib>:"Add State(s) to Queue__jki_lib_state_machine.vi"("State(s) in Front (\"\")"="/* Post Error States", "State(s) in (\"\")"=w103) -> ("States Out"=w102:string)  [unwired: 13 in]
      }
      frame "Exit" {
        # "Do not put any code in this frame.\n(No errors that occur here will be handled.)"
        n41 = call <vilib>:"Add State(s) to Queue__jki_lib_state_machine.vi"("State(s) in (\"\")"=w108) -> ("States Out"=w107:string)  [unwired: 14 in]
      }
      frame "---------- Data ----------" {
        # "Do not put any code in this frame.\n(It is a separator no-op. You can make a copy of this frame to create a new Data frame)"
        n42 = call <vilib>:"Add State(s) to Queue__jki_lib_state_machine.vi"("State(s) in (\"\")"=w112) -> ("States Out"=w111:string)  [unwired: 14 in]
      }
      frame "Data: Initialize" {
        w113 = string[][] []  # Temporary Preset
        w117 = T5 {"Current VI Reference"=refnum, "Close Panel on Exit?"=FALSE}  # Core
        w119 = TRUE  # Your Boolean data
        w118 = ""  # Your string data
        # "do not delete - used by framework"
        # "Expand Bundle to add new data elements to shift register data."
        # "Add new data here."
        # "Data names and types of shift register data are defined by this bundle."
        # "Initialize the shift-register data, here.\n(data names are defined by what you wire into the bundle function)"
        n43 = property on="Headers" class="Tbl (strict)"() -> ("Column Headers[]"=w114:string[])  [unwired: 2 in, 2 out]
        n44 = Bundle("Core"=w117, "Your Boolean data"=w119, "Your string data"=w118, "Table Control"="Table Control", "Column Headers[]"=w114, "Temporary Preset"=w113) -> (w116:T4)  [unwired: 1 in]
        n45 = call <vilib>:"Add State(s) to Queue__jki_lib_state_machine.vi"("State(s) in (\"\")"=w122) -> ("States Out"=w121:string)  [unwired: 14 in]
      }
      frame "Data: Cleanup" {
        # "Cleanup any data and references, here.\n(this is called automatically, by the Macro: Exit)"
        n46 = Unbundle By Name(w123) -> ("Core.Current VI Reference"=w126:refnum<vi>)
        n47 = Close Reference(reference=w126, error in (no error)=w125) -> (error out=w124:errorcluster)
        n48 = call <vilib>:"Add State(s) to Queue__jki_lib_state_machine.vi"("State(s) in (\"\")"=w128) -> ("States Out"=w127:string)  [unwired: 14 in]
      }
      frame "---------- UI ----------" {
        # "Do not put any code in this frame.\n(It is a separator no-op. You can make a copy of this frame to create a new UI frame)"
        n49 = call <vilib>:"Add State(s) to Queue__jki_lib_state_machine.vi"("State(s) in (\"\")"=w132) -> ("States Out"=w131:string)  [unwired: 14 in]
      }
      frame "UI: Initialize" {
        # "Initialize the User Interface, here.\n(this is called automatically, by the Macro: Init)"
        n50 = call <vilib>:"Add State(s) to Queue__jki_lib_state_machine.vi"("State(s) in (\"\")"=w136) -> ("States Out"=w135:string)  [unwired: 14 in]
      }
      frame "UI: Cursor Set" {
        # "Argument"
        # "Set and Unset Cursor Busy.\n(Usage: \"UI: Cursor Set >> Busy|Idle\")"
        n51 = case shown="\"Idle\", Default" w137 {
          tunnel: w139 -> [w144 w146]
          tunnel: [w143 w145] -> w138
          frame "Idle", Default {
            n52 = call <vilib>:"Unset Busy.vi"("error in (no error)"=w144) -> ("error out"=w143:errorcluster)  [unwired: 10 in]
          }
          frame "Busy" {
            n53 = call <vilib>:"Set Busy.vi"("error in (no error)"=w146) -> ("error out"=w145:errorcluster)  [unwired: 9 in, 1 out]
          }
        }
        n54 = call <vilib>:"Add State(s) to Queue__jki_lib_state_machine.vi"("State(s) in (\"\")"=w142) -> ("States Out"=w141:string)  [unwired: 14 in]
      }
      frame "UI: Front Panel State" {
        # "Argument"
        # "Set Front Panel Open or Closed\n(Usage: \"UI: Front Panel State >> Open|Close\")"
        n55 = Unbundle By Name(w149) -> ("Core.Current VI Reference"=w148:refnum<vi>)
        n56 = case shown="\"Minimize\", \"Minimized\"" w147 {
          tunnel: w151 -> [w159 w174 w185 w198 w211]
          tunnel: [w161 w175 w187 w200 w213] -> w150
          tunnel: w148 -> [w160 w172 w186 w199 w212]
          frame "Open", "Standard", Default {
            w154 = T2."Standard" ("State")
            n57 = property class="VI"(reference=w160, error in=w159) -> (reference out=w157:refnum<vi>, error out=w158:errorcluster, "FP.State"=w156:T2)
            n58 = Not Equal?(x=w156, y=w154) -> (x != y?=w155:bool)
            n59 = case shown="True" w155 {
              tunnel: [w165 w167] -> w161
              tunnel: w158 -> [w164 w167]
              tunnel: w157 -> [w163 _]
              tunnel: w154 -> [w162 _]
              frame True {
                n60 = invoke class="VI" method="FP.Open"(reference=w163, error in=w164, "Activate"=TRUE, "State"=w162) -> (error out=w165:errorcluster)  [unwired: 1 in, 4 out]
              }
              frame False {
              }
            }
          }
          frame "Close", "Closed" {
            n61 = property class="VI"(reference=w172, error in=w174) -> (reference out=w171:refnum<vi>, error out=w173:errorcluster, "FP.State"=w169:T2)
            n62 = Not Equal?(x=w169, y=T2."Closed" ("Front Panel Window:State")) -> (x != y?=w168:bool)
            n63 = case shown="True" w168 {
              tunnel: [w176 w179] -> w175
              tunnel: w173 -> [w176 w178]
              tunnel: w171 -> [_ w177]
              frame False {
              }
              frame True {
                n64 = invoke class="VI" method="FP.Close"(reference=w177, error in=w178) -> (error out=w179:errorcluster)  [unwired: 1 in, 2 out]
              }
            }
          }
          frame "Hidden", "Hide" {
            w180 = T2."Hidden" ("State")
            n65 = property class="VI"(reference=w186, error in=w185) -> (reference out=w183:refnum<vi>, error out=w184:errorcluster, "FP.State"=w182:T2)
            n66 = Not Equal?(x=w182, y=w180) -> (x != y?=w181:bool)
            n67 = case shown="True" w181 {
              tunnel: [w191 w192] -> w187
              tunnel: w184 -> [w190 w192]
              tunnel: w183 -> [w189 _]
              tunnel: w180 -> [w188 _]
              frame True {
                n68 = invoke class="VI" method="FP.Open"(reference=w189, error in=w190, "State"=w188) -> (error out=w191:errorcluster)  [unwired: 2 in, 4 out]
              }
              frame False {
              }
            }
          }
          frame "Minimize", "Minimized" {
            w193 = T2."Minimized" ("State")
            n69 = property class="VI"(reference=w199, error in=w198) -> (reference out=w196:refnum<vi>, error out=w197:errorcluster, "FP.State"=w195:T2)
            n70 = Not Equal?(x=w195, y=w193) -> (x != y?=w194:bool)
            n71 = case shown="True" w194 {
              tunnel: [w204 w205] -> w200
              tunnel: w197 -> [w203 w205]
              tunnel: w196 -> [w202 _]
              tunnel: w193 -> [w201 _]
              frame True {
                n72 = invoke class="VI" method="FP.Open"(reference=w202, error in=w203, "State"=w201) -> (error out=w204:errorcluster)  [unwired: 2 in, 4 out]
              }
              frame False {
              }
            }
          }
          frame "Maximize", "Maximized" {
            w206 = T2."Maximized" ("State")
            n73 = property class="VI"(reference=w212, error in=w211) -> (reference out=w209:refnum<vi>, error out=w210:errorcluster, "FP.State"=w208:T2)
            n74 = Not Equal?(x=w208, y=w206) -> (x != y?=w207:bool)
            n75 = case shown="True" w207 {
              tunnel: [w217 w218] -> w213
              tunnel: w210 -> [w216 w218]
              tunnel: w209 -> [w215 _]
              tunnel: w206 -> [w214 _]
              frame True {
                n76 = invoke class="VI" method="FP.Open"(reference=w215, error in=w216, "State"=w214) -> (error out=w217:errorcluster)  [unwired: 2 in, 4 out]
              }
              frame False {
              }
            }
          }
        }
        n77 = call <vilib>:"Add State(s) to Queue__jki_lib_state_machine.vi"("State(s) in (\"\")"=w153) -> ("States Out"=w152:string)  [unwired: 14 in]
      }
      frame "---------- Macro ----------" {
        # "Do not put any code in this frame.\n(It is a separator no-op. You can make a copy of this frame to create a new Macro frame)"
        n78 = call <vilib>:"Add State(s) to Queue__jki_lib_state_machine.vi"("State(s) in (\"\")"=w222) -> ("States Out"=w221:string)  [unwired: 14 in]
      }
      frame "Macro: Initialize" {
        w223 = "Data: Initialize\nInitialize Core Data\nUI: Initialize\nUI: Front Panel State >> Open"  # Data: Initialize Initialize Core Data UI: Initialize UI: Front Panel State >> Open
        # "Initialization Macro\n(This is called once, when the VI starts)"
        n79 = call <vilib>:"Add State(s) to Queue__jki_lib_state_machine.vi"("State(s) in Front (\"\")"=w223, "State(s) in (\"\")"=w227) -> ("States Out"=w226:string)  [unwired: 13 in]
      }
      frame "Macro: Exit" {
        # "Exit Macro\n(This is called once, when the VI exits)"
        n80 = Unbundle By Name(w234) -> ("Core.Close Panel on Exit?"=w233:bool)
        n81 = Select(t="UI: Front Panel State >> Close", s=w233, f="") -> (s? t:f=w230:string)
        n82 = call <vilib>:"Add State(s) to Queue__jki_lib_state_machine.vi"("State(s) in (\"\")"=w230, "State(s) at Back (\"\")"="Data: Cleanup\nExit") -> ("States Out"=w228:string)  [unwired: 13 in]
        n83 = call <vilib>:"Add State(s) to Queue__jki_lib_state_machine.vi"("State(s) in Front (\"\")"=w228, "State(s) in (\"\")"=w237) -> ("States Out"=w236:string)  [unwired: 13 in]
      }
      frame "---------- New Category ----------" {
        # "Template Separator\n(You can make a copy of, or modify, this frame)"
        n84 = call <vilib>:"Add State(s) to Queue__jki_lib_state_machine.vi"("State(s) in (\"\")"=w241) -> ("States Out"=w240:string)  [unwired: 14 in]
      }
      frame "Compare Table" {
        # "Template Separator\n(You can make a copy of, or modify, this frame)"
        n85 = property on="PRESET FROM DB" class="Tbl (strict)"() -> ("Value"=w248:string[][])  [unwired: 2 in, 2 out]
        n86 = property on="ECS File" class="Tbl (strict)"() -> ("Value"=w247:string[][])  [unwired: 2 in, 2 out]
        n87 = call "Left Join.vi"("Array 2"=w247, "Array 1"=w248) -> ("Left Joined Array"=w245:string[][])  [unwired: 9 in]
        n88 = call <vilib>:"Add State(s) to Queue__jki_lib_state_machine.vi"("State(s) in Front (\"\")"="Table Update" ("State(s) in Front (\"\")"), "State(s) in (\"\")"=w251) -> ("States Out"=w250:string)  [unwired: 13 in]
        n89 = Bundle By Name(cluster=w246, "Table Control"=w245, "Column Headers[]"=string[] ["Device Name", "Device Variable", "Preset Value", "ECS Value"] ("Column Headers")) -> (w244:T4)
      }
      frame "Choose Values" {
        # "Template Separator\n(You can make a copy of, or modify, this frame)"
        n90 = property on="Table Control" class="Tbl (strict)"() -> ("Value"=w255:string[][])  [unwired: 2 in, 2 out]
        n91 = call "Value_Selection_in_Table_GUI.vi"("Column Headers"=string[] ["Device Name", "Device Variable", "Preset Value", "ECS Value"], "SELECTION TABLE - Click on values to keep"=w255) -> ("Coordinate Array"=→"Coordinate Array":i32[][])  [unwired: 9 in]
        n92 = call <vilib>:"Add State(s) to Queue__jki_lib_state_machine.vi"("State(s) in Front (\"\")"="Implement Value Change" ("State(s) in Front (\"\")"), "State(s) in (\"\")"=w259) -> ("States Out"=w258:string)  [unwired: 13 in]
      }
      frame "Implement Value Change" {
        # "Template Separator\n(You can make a copy of, or modify, this frame)"
        n93 = Unbundle By Name(w265) -> ("Table Control"=w263:string[][])
        n94 = property on="Coordinate Array" class="Arr (strict)"() -> ("Value"=w262:i32[][])  [unwired: 2 in, 2 out]
        n95 = call "Value_Update_to_Preset.vi"("Coordinate Array with Changes"=w262, "Input Table"=w263) -> ("Column Headers"=w260:string[], "Output Table with Changes"=w261:string[][])  [unwired: 8 in]
        n96 = Bundle By Name(cluster=w265, "Table Control"=w261, "Column Headers[]"=w260) -> (w264:T4)
        n97 = call <vilib>:"Add State(s) to Queue__jki_lib_state_machine.vi"("State(s) in Front (\"\")"="Table Update" ("State(s) in Front (\"\")"), "State(s) in (\"\")"=w269) -> ("States Out"=w268:string)  [unwired: 13 in]
      }
      frame "Load Preset from DB" {
        # "Template Separator\n(You can make a copy of, or modify, this frame)"
        n98 = property on="Preset Menu" class="Ring (strict)"() -> ("RingText.Text"=w275:string)  [unwired: 2 in, 2 out]
        n99 = call "preset SQL Queries.vi"("Expt name / MCIP/ Variable/Preset Name"=w275, "Preset Query"=Preset_Query_Enum."GetPresetDeviceNames") -> ("data"=w278:string[][])  [unwired: 7 in, 2 out]
        n100 = Array Subset(array=w278, index (row)=1 ("index")) -> (w276:string[][])  [unwired: 3 in]
        n101 = for {
          tunnel: w276 -> [w286] mode=indexing
          tunnel: w275 -> [w287]
          tunnel: [w283] -> w271 mode=concatenating
          n102 = Index Array(array=w286) -> (element=w284:string)  [unwired: 1 in]
          n103 = call "preset SQL Queries.vi"("Expt name / MCIP/ Variable/Preset Name"=w287, "Device/Devicetype name\n/Plotter.id/ScanName#"=w284, "Preset Query"=Preset_Query_Enum."GetDevicePresetVariables") -> ("data"=w289:string[][])  [unwired: 6 in, 2 out]
          n104 = Array Subset(array=w289, index (row)=1 ("index")) -> (w285:string[][])  [unwired: 3 in]
          n105 = for {
            tunnel: w285 -> [w296] mode=indexing
            tunnel: [w295] -> w283 mode=indexing
            tunnel: w284 -> [w292]
            n106 = Index Array(array=w296, index=0 ("index (row)")) -> (element=w294:string)
            n107 = Index Array(array=w296, index=1 ("disabled index (col)")) -> (element=w293:string)
            n108 = Wait (ms)(milliseconds to wait=u32 20) -> ()  [unwired: 1 out]
            n109 = Build Array(w292, w294, w293) -> (w295:string[])
          }
        }
        "PRESET FROM DB" <- w271
        n110 = Bundle By Name(cluster=w274, "Table Control"=w271, "Column Headers[]"=string[] ["Device Name", "Device Variable", "Preset Value"] ("Column Headers")) -> (w273:T4)
        n111 = call <vilib>:"Add State(s) to Queue__jki_lib_state_machine.vi"("State(s) in Front (\"\")"="Table Update" ("State(s) in Front (\"\")"), "State(s) in (\"\")"=w282) -> ("States Out"=w281:string)  [unwired: 13 in]
      }
      frame "Load Configuration File" {
        # "Template Separator\n(You can make a copy of, or modify, this frame)"
        n112 = call "Configuration_to_Array.vi"("file (use dialog)"="file (use dialog)") -> ("Table Control"=w301:string[][])  [unwired: 10 in]
        "ECS File" <- w301
        n113 = Bundle By Name(cluster=w303, "Table Control"=w301, "Column Headers[]"=string[] ["Device Name", "Device Variable", "ECS Values"] ("Column Headers")) -> (w302:T4)
        n114 = call <vilib>:"Add State(s) to Queue__jki_lib_state_machine.vi"("State(s) in Front (\"\")"="Table Update" ("State(s) in Front (\"\")"), "State(s) in (\"\")"=w307) -> ("States Out"=w306:string)  [unwired: 13 in]
      }
      frame "Upload Preset" {
        # "Template Separator\n(You can make a copy of, or modify, this frame)"
        n115 = call <vilib>:"Three Button Dialog.vi"("Right Button Text (\"Cancel\")"="Cancel" ("Right Button Text (\"Cancel\")"), "Center Button Text (\"No\")"="Overwrite Existing Preset" ("Right Button Text (\"Cancel\")"), "Left Button Text (\"Yes\")"="Save as New Preset" ("Left Button Text (\"Yes\")"), "message"="Save the current preset as - ") -> ("Which Button?"=w309:T6)  [unwired: 7 in]
        n116 = case shown="\"Center Button\"" w309 {
          tunnel: ["Save as New Preset" ("State(s) in Front (\"\")") "Overwrite Existing Preset" ("Right Button Text (\"Cancel\")")] -> w308
          frame "Left Button", Default {
          }
          frame "Center Button" {
          }
        }
        n117 = call <vilib>:"Add State(s) to Queue__jki_lib_state_machine.vi"("State(s) in Front (\"\")"=w308, "State(s) in (\"\")"=w317) -> ("States Out"=w316:string)  [unwired: 13 in]
      }
      frame "Save as New Preset" {
        # "Template Separator\n(You can make a copy of, or modify, this frame)"
        n118 = call "Preset Name"() -> ("Name"=w326:string, "OK"=w329:bool)  [unwired: 17 in, 1 out]
        n119 = property on="Preset Menu" class="Ring (strict)"() -> ("Strings []"=w325:string[])  [unwired: 2 in, 2 out]
        n120 = Search 1D Array(1D array=w325, element=w326) -> (index of element=w324:i32)  [unwired: 1 in]
        n121 = call <vilib>:"Trim Whitespace.vi"("string"=w326) -> ("trimmed string"=w328:string)  [unwired: 1 in]
        n122 = Equal?(x=w328, y="") -> (x = y?=w322:bool)
        n123 = Not Equal?(x=w324, y=-1) -> (x != y?=w321:bool)
        n124 = Or(x=w322, y=w321) -> (x .or. y?=w320:bool)
        n125 = case shown="True" w329 {
          tunnel: w320 -> [_ w335]
          frame False {
          }
          frame True {
            n126 = case shown="False" w335 {
              frame False {
              }
              frame True {
                n127 = One Button Dialog(message="Name field was blank or the Preset Name already exists") -> ()  [unwired: 1 in, 1 out]
              }
            }
          }
        }
        n128 = call <vilib>:"Add State(s) to Queue__jki_lib_state_machine.vi"("State(s) in Front (\"\")"="Table Update" ("State(s) in Front (\"\")"), "State(s) in (\"\")"=w334) -> ("States Out"=w333:string)  [unwired: 13 in]
      }
      frame "Overwrite Existing Preset" {
        # "Template Separator\n(You can make a copy of, or modify, this frame)"
        n129 = property on="Preset Menu" class="Ring (strict)"() -> ("RingText.Text"=w341:string)  [unwired: 2 in, 2 out]
        n130 = Concatenate Strings("Are you sure you want to overwrite " ("string"), w341, " with the current table ?" ("string")) -> (w339:string)
        n131 = Two Button Dialog(message=w339, 2:"Yes" ("T button name (\"OK\")")) -> (T button?=w337:bool)  [unwired: 1 in]
        n132 = case shown="True" w337 {
          frame False {
          }
          frame True {
          }
        }
        n133 = call <vilib>:"Add State(s) to Queue__jki_lib_state_machine.vi"("State(s) in Front (\"\")"="Table Update" ("State(s) in Front (\"\")"), "State(s) in (\"\")"=w347) -> ("States Out"=w346:string)  [unwired: 13 in]
      }
      frame "New Category: 1" {
        # "Your code here.\n(You can make a copy of, or modify, this frame)"
        n134 = call <vilib>:"Add State(s) to Queue__jki_lib_state_machine.vi"("State(s) in (\"\")"=w351) -> ("States Out"=w350:string)  [unwired: 14 in]
      }
      frame "New Category: 2" {
        # "Your code here.\n(You can make a copy of, or modify, this frame)"
        n135 = call <vilib>:"Add State(s) to Queue__jki_lib_state_machine.vi"("State(s) in (\"\")"=w355) -> ("States Out"=w354:string)  [unwired: 14 in]
      }
      frame "-------Table Update--------" {
        # "Template Separator\n(You can make a copy of, or modify, this frame)"
        n136 = call <vilib>:"Add State(s) to Queue__jki_lib_state_machine.vi"("State(s) in (\"\")"=w359) -> ("States Out"=w358:string)  [unwired: 14 in]
      }
      frame "Table Update" {
        # "Template Separator\n(You can make a copy of, or modify, this frame)"
        n137 = Unbundle By Name(w362) -> ("Table Control"=w361:string[][], "Column Headers[]"=w360:string[])
        n138 = call <vilib>:"Add State(s) to Queue__jki_lib_state_machine.vi"("State(s) in (\"\")"=w365) -> ("States Out"=w364:string)  [unwired: 14 in]
        n139 = property on="Table Control" class="Tbl (strict)"("Value"=w361, "Column Headers[]"=w360) -> ()  [unwired: 2 in, 2 out]
      }
    }
  }
